vi "Create CAN Incoming Section.vi"(8 "error in (no error)":errorcluster, 11 "Device Item Ref in":T1 format="%.0x") -> (0 "error out":errorcluster, 3 "Device Item Ref Out":T1=18446744073709551615 format="%.0x")   [LabVIEW 2015, in "J1939 Addon Shared.lvlib"]
uses:
  J1939 Addon Shared.lvlib
  <vilib>/NI Veristand/Custom Device API/Custom Device Item Ref.ctl
  Constants.vi
  <vilib>/NI/NIVS System Definition Utilities/System Definition Utilities.lvlib
  <vilib>/NI VeriStand/Custom Device API/Custom Device API.lvlib
panel:
  # "OUTPUTS"
  # "INPUTS"
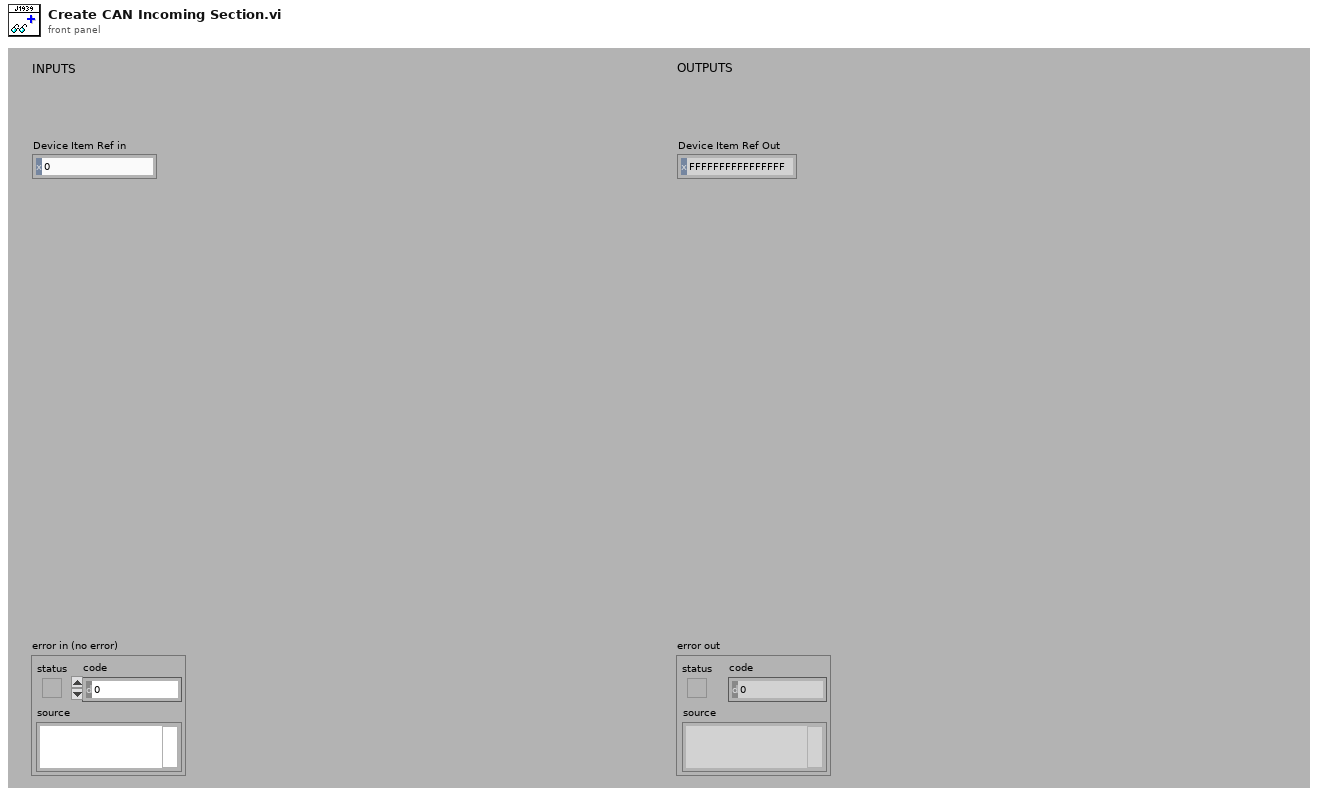
[diagram p1: front panel]
types:
  T1 = typedef "Custom Device API.lvlib/Custom Device Item Ref.ctl" = u64
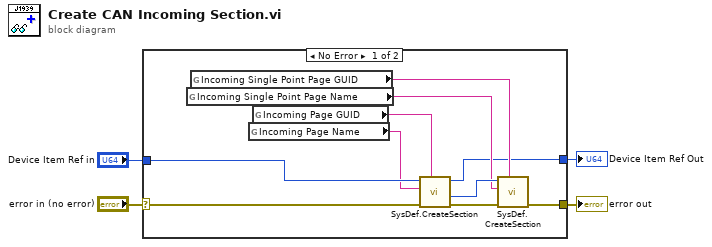
[diagram p0: block diagram]
diagram:
  n1 = case shown="No Error" "error in (no error)" {
    selector: "error in (no error)" -> [w13 w16]
    tunnel: [w10 w16] -> w3
    tunnel: "Device Item Ref in" -> [w14 w15]
    tunnel: [w5 w15] -> w1
    frame No Error {
      n2 = global read "Constants.vi" "Incoming Single Point Page Name"() -> (w6:string)
      n3 = global read "Constants.vi" "Incoming Single Point Page GUID"() -> (w7:string)
      n4 = global read "Constants.vi" "Incoming Page Name"() -> (w8:string)
      n5 = global read "Constants.vi" "Incoming Page GUID"() -> (w9:string)
      n6 = call <vilib>:"SysDef.CreateSection.vi"("GUID"=w9, "error in (no error)"=w13, "Name"=w8, "nodeID"=w14) -> ("error out"=w12:errorcluster, "New NodeID"=w11:u64, "nodeID out"=w5:u64)  [unwired: 4 in, 1 out]
      n7 = call <vilib>:"SysDef.CreateSection.vi"("GUID"=w7, "error in (no error)"=w12, "Name"=w6, "nodeID"=w11) -> ("error out"=w10:errorcluster)  [unwired: 4 in, 3 out]
    }
    frame Error {
    }
  }
  "error out" <- w3
  "Device Item Ref Out" <- w1
